vi "PCO_SetConfig.vi"(8 "error in":errorcluster caption="entrée d'erreur", 11 "PCO_Config":T1 {"TriggerMode" items=["auto sequence", "software trigger", "external exposure start", "external exposure control"]}) -> (0 "error out":errorcluster caption="sortie d'erreur", 1 "PCO_Config 2":T1 {"TriggerMode" items=["auto sequence", "software trigger", "external exposure start", "external exposure control"]}, 2 "Trigger externe?":bool, 3 "configuration":T3 {"binning"."mode" items=["sum", "average"]})   [LabVIEW 2026]
uses:
  <instrlib>/PCO_SDK/File Group 0/vi.lib/Excelitas PCO GmbH/pco.labview/camera/Controls/binning.ctl
  Controls/PCO_Config.ctl
  <instrlib>/PCO_SDK/File Group 0/vi.lib/Excelitas PCO GmbH/pco.labview/camera/Camera.lvclass
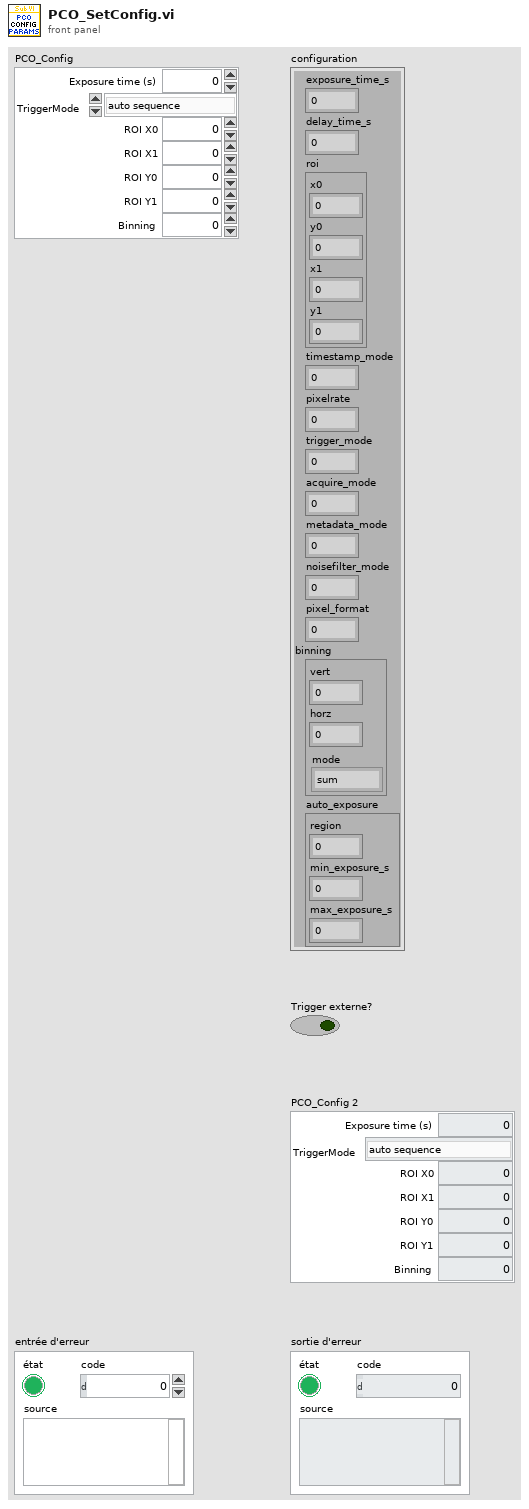
[diagram p1: front panel]
types:
  T1 = typedef "PCO_Config.ctl" = cluster{"Exposure time (s)":dbl, "TriggerMode":u16, "ROI X0":u16, "ROI Y0":u16, "ROI X1":u16, "ROI Y1":u16, "Binning":u8}
  T2 = typedef "Camera.lvclass/binning.ctl" = cluster{"vert":u16, "horz":u16, "mode":u16}
  T3 = cluster{"exposure_time_s":dbl, "delay_time_s":dbl, "roi":cluster{"x0":u64, "y0":u64, "x1":u64, "y1":u64}, "timestamp_mode":u16, "pixelrate":u32, "trigger_mode":u16, "acquire_mode":u16, "metadata_mode":u16, "noisefilter_mode":u16, "pixel_format":u32, "binning":T2, "auto_exposure":cluster{"region":u16, "min_exposure_s":dbl, "max_exposure_s":dbl}}
  T4 = enum16{"auto sequence", "software trigger", "external exposure start", "external exposure control"}
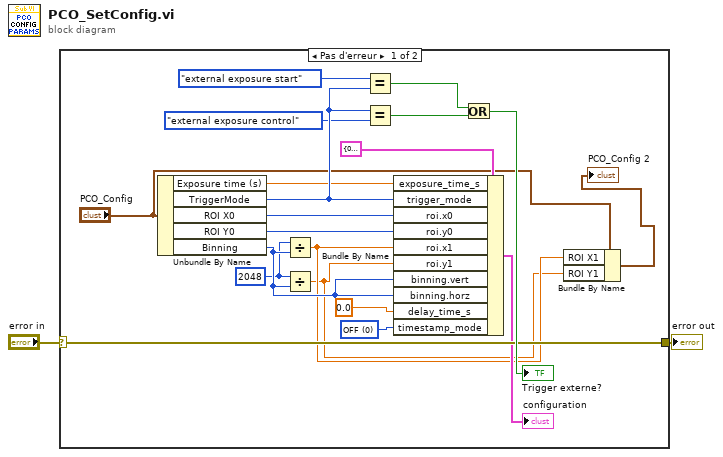
[diagram p0: block diagram]
diagram:
  n1 = case shown="Pas d'erreur" "error in" {
    selector: "error in" -> [w10 w23]
    tunnel: [w10 w23] -> w1
    frame No Error {
      w7 = 2048
      w14 = u16 0 items=["OFF", "Binary", "Binary+ASCII", "ASCII"] ("wTimeStampMode")
      n2 = Unbundle By Name("PCO_Config") -> ("Exposure time (s)"=w12:dbl, "TriggerMode"=w21:u16, "ROI X0"=w15:u16, "ROI Y0"=w16:u16, "Binning"=w9:u8)
      n3 = Divide(x=w7, y=w9) -> (x/y=w4:dbl)
      n4 = Divide(x=w7, y=w9) -> (x/y=w3:dbl)
      n5 = Equal?(x=T4."external exposure start" ("TriggerMode"), y=w21) -> (x = y?=w19:bool)
      n6 = Equal?(x=w21, y=T4."external exposure control" ("TriggerMode")) -> (x = y?=w20:bool)
      n7 = Bundle By Name(cluster=T3 {"exposure_time_s"=0.1, "delay_time_s"=nan, "roi"={"x0"=18446744073709551615, "y0"=18446744073709551615, "x1"=18446744073709551615, "y1"=18446744073709551615}, "timestamp_mode"=65535, "pixelrate"=4294967295, "trigger_mode"=65535, "acquire_mode"=65535, "metadata_mode"=65535, "noisefilter_mode"=65535, "pixel_format"=4294967295, "binning"={"vert"=65535, "horz"=65535, "mode"=0}, "auto_exposure"={"region"=0, "min_exposure_s"=0.001, "max_exposure_s"=0.1}} ("configuration"), "exposure_time_s"=w12, "trigger_mode"=w21, "roi.x0"=w15, "roi.y0"=w16, "roi.x1"=w4, "roi.y1"=w3, "binning.vert"=w9, "binning.horz"=w9, "delay_time_s"=0.0, "timestamp_mode"=w14) -> (→"configuration":T3)
      n8 = Or(x=w19, y=w20) -> (x .or. y?=→"Trigger externe?":bool)
      n9 = Bundle By Name(cluster="PCO_Config", "ROI X1"=w4, "ROI Y1"=w3) -> (→"PCO_Config 2":T1)
    }
    frame Error {
    }
  }
  "error out" <- w1
